vi "Set Up Terminal for Input Param.vi"(6 "ConPane Terminal Index":u32, 7 "CallLibrary Terminal Index":i32, 9 "CalllLibrary Ref":refnum<vi>, 10 "VI Ref":refnum<vi>, 11 "Enum Writer in":refnum<class "Enum Writer.lvclass">) -> (3 "Enum Writer out":refnum<class "Enum Writer.lvclass">)   [LabVIEW 2013, in "Enum Writer.lvclass"]
uses:
  Enum Writer.lvclass
  Enum Writer.lvclass/Enum Writer.ctl
  Abstract Param Writer/Abstract Param Writer.lvclass
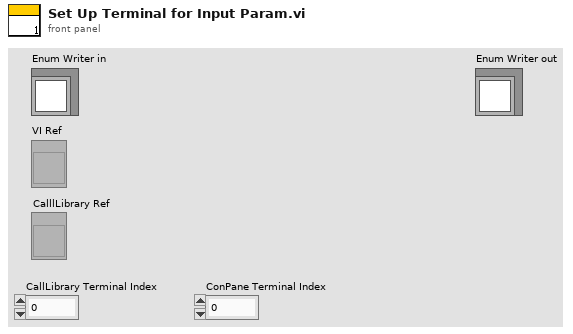
[diagram p1: front panel]
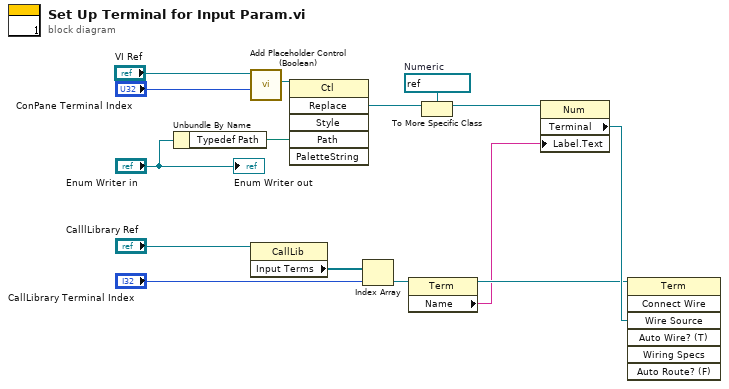
[diagram p0: block diagram]
diagram:
  w14 = refnum<vi> refnum  # Numeric
  n1 = Unbundle By Name("Enum Writer in") -> ("Typedef Path"=w1:path)
  n2 = call "Add Placeholder Control (Boolean).vi"("ConPane Terminal Index"="ConPane Terminal Index", "VI Ref"="VI Ref") -> ("Control Ref"=w15:refnum<vi>)  [unwired: 9 in]
  n3 = property class="CallLib"(reference="CalllLibrary Ref") -> ("Input Terms"=w11:refnum<vi>[])  [unwired: 1 in, 2 out]
  n4 = invoke class="Ctl" method="Replace"(reference=w15, "Path"=w1) -> ("Replace"=w8:refnum<vi>)  [unwired: 4 in, 5 out]
  n5 = Index Array(array=w11, index="CallLibrary Terminal Index") -> (element=w12:refnum<vi>)
  n6 = property class="Term"(reference=w12) -> (reference out=w9:refnum<vi>, "Name"=w7:string)  [unwired: 1 in, 1 out]
  n7 = To More Specific Class(target class=w14, reference=w8) -> (specific class reference=w13:refnum<vi>)  [unwired: 1 in, 1 out]
  n8 = property class="Num"(reference=w13, "Label.Text"=w7) -> ("Terminal"=w10:refnum<vi>)  [unwired: 1 in, 2 out]
  n9 = invoke class="Term" method="Connect Wire"(reference=w9, "Wire Source"=w10) -> ()  [unwired: 5 in, 7 out]
  "Enum Writer out" <- "Enum Writer in"
